vi "Get Attributes Priv.vi"(0 "Tree Dictionary In":variant, 5 "Unique ID":string, 7 "Name":string, 11 "error in":errorcluster) -> (4 "Tree Dictionary Out":variant, 6 "Found?":bool, 8 "Data":variant, 15 "error out":errorcluster)   [LabVIEW 2016, in "Tree Manager.lvclass"]
uses:
  Tree Manager.lvclass
  Typedefs/Tree.ctl
  <vilib>/Utility/error.llb/Error Cluster From Error Code.vi
  <vilib>/ErrorRing/Error Ring.xnode
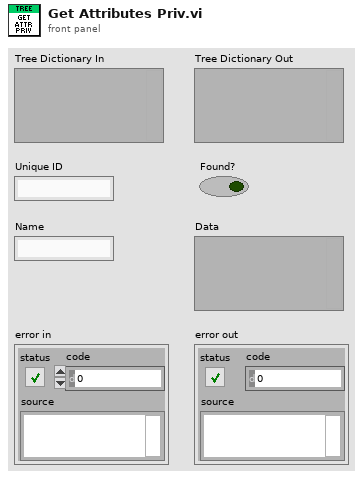
[diagram p1: front panel]
types:
  T1 = typedef "Tree Manager.lvclass/Tree.ctl" = cluster{"Unique ID":string, "Parent ID":string, "Child IDs":string[], "Data":variant, "Name":string}
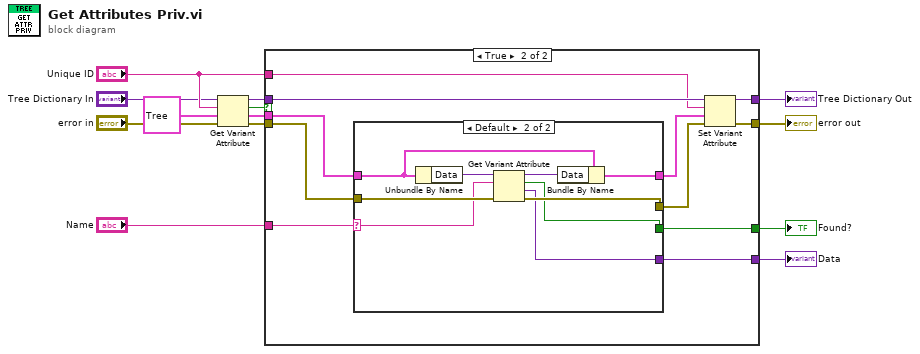
[diagram p0: block diagram]
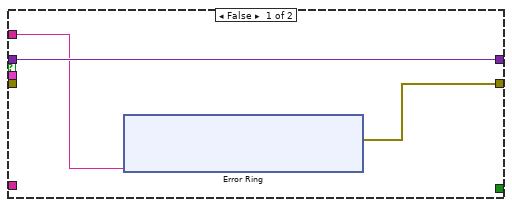
[diagram p2: hidden frame]
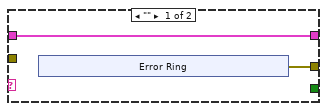
[diagram p3: hidden frame]
diagram:
  n1 = Get Variant Attribute(Variant="Tree Dictionary In", name="Unique ID", default value (empty Variant)=T1 {"Unique ID"="", "Parent ID"="", "Child IDs"=[], "Data"=variant, "Name"=""} ("Cluster of class private data"), error in="error in") -> (duplicate Variant=w7:variant, found=w8:bool, value=w9:T1, error out=w5:errorcluster)
  n2 = case shown="True" w8 {
    tunnel: [w15 w34] -> w3
    tunnel: [w16 w33] -> w4
    tunnel: w5 -> [_ w30]
    tunnel: w7 -> [w16 w32]
    tunnel: w9 -> [_ w24]
    tunnel: "Name" -> [_ w28]
    tunnel: "Unique ID" -> [w14 w25]
    tunnel: [_ w27] -> w10
    tunnel: [_ w26] -> w11
    frame False {
      n3 = xnode "Error Ring"("parameter 0"=w14) -> ("error out"=w15:errorcluster)
    }
    frame True {
      n4 = case shown="Default" w28 {
        selector: w28 -> [_ w46]
        tunnel: [w35 w49] -> w31
        tunnel: w30 -> [_ w48]
        tunnel: [w36 w47] -> w29
        tunnel: [_ w45] -> w27
        tunnel: [_ w44] -> w26
        tunnel: w24 -> [w35 w42]
        frame "" {
          n5 = xnode "Error Ring"() -> ("error out"=w36:errorcluster)
        }
        frame Default {
          n6 = Unbundle By Name(w42) -> ("Data"=w43:variant)
          n7 = Get Variant Attribute(Variant=w43, name=w46, error in=w48) -> (duplicate Variant=w50:variant, found=w45:bool, value=w44:variant, error out=w47:errorcluster)  [unwired: 1 in]
          n8 = Bundle By Name(cluster=w42, "Data"=w50) -> (w49:T1)
        }
      }
      n9 = Set Variant Attribute(Variant=w32, name=w25, value=w31, error in=w29) -> (Variant out=w33:variant, error out=w34:errorcluster)  [unwired: 1 out]
    }
  }
  "Data" <- w11
  "Found?" <- w10
  "Tree Dictionary Out" <- w4
  "error out" <- w3
